vi "EXA_Instrument_Mode.vi"(8 "error in":errorcluster, 10 "Mode":enum16{"SA", "LTE"}(ring), 11 "VISA resource name":refnum<visa-resource-name>) -> (0 "error out":errorcluster, 3 "VISA resource name":refnum<visa-resource-name>)   [LabVIEW 2016]
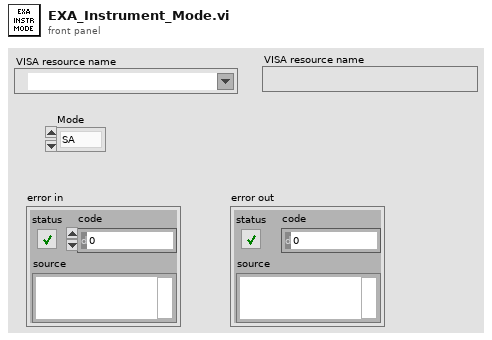
[diagram p1: front panel]
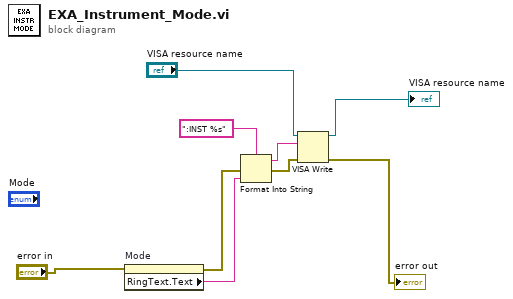
[diagram p0: block diagram]
diagram:
  n1 = property on="Mode" class="Enum (strict)"(error in="error in") -> (error out=w5:errorcluster, "RingText.Text"=w3:string)  [unwired: 1 in, 1 out]
  n2 = Format Into String(format string=":INST %s", error in=w5, w3) -> (resulting string=w1:string, error out=w7:errorcluster)  [unwired: 1 in]
  n3 = VISA Write(VISA resource name="VISA resource name", write buffer=w1, error in (no error)=w7) -> (VISA resource name out=→"VISA resource name":refnum<visa-resource-name>, error out=→"error out":errorcluster)  [unwired: 1 out]
